vi "generate_jv_filepath.vi"(6 "Light or dark":string, 9 "Pixel":string, 10 "Cell Label":string, 11 "Data Output Folder":path) -> (2 "Scan number":string, 3 "File path":path)   [LabVIEW 2016]
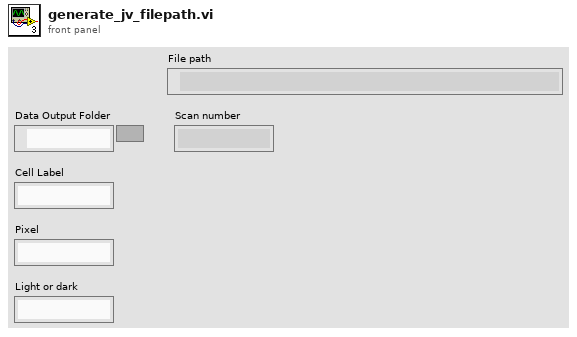
[diagram p1: front panel]
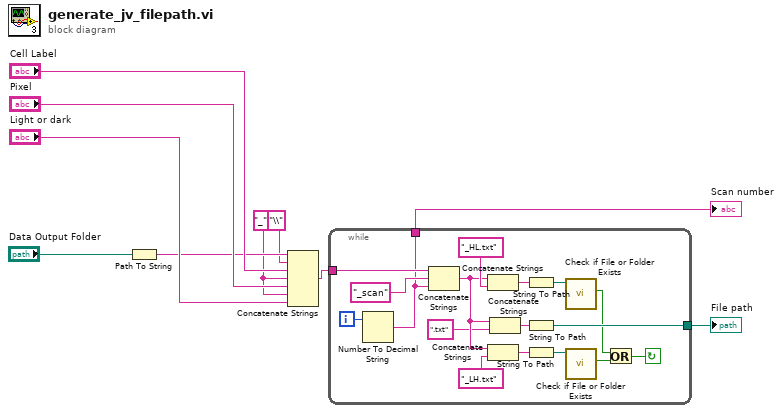
[diagram p0: block diagram]
diagram:
  w2 = "_"
  n1 = Path To String(path="Data Output Folder") -> (string=w4:string)
  n2 = Concatenate Strings(w4, "\\", "Cell Label", w2, "Pixel", w2, "Light or dark") -> (w5:string)
  n3 = while {
    tunnel: w5 -> [w27]
    tunnel: [w24] -> w9
    tunnel: [w18] -> w1
    i -> [w23]
    stop <- w14 continue-if-true
    n4 = Number To Decimal String(number=w23) -> (decimal integer string=w24:string)  [unwired: 1 in]
    n5 = Concatenate Strings(w27, "_scan", w24) -> (w13:string)
    n6 = Concatenate Strings(w13, "_HL.txt") -> (w22:string)
    n7 = Concatenate Strings(w13, "_LH.txt") -> (w19:string)
    n8 = Concatenate Strings(w13, ".txt" ("string")) -> (w11:string)
    n9 = String To Path(string=w22) -> (path=w25:path)
    n10 = String To Path(string=w11) -> (path=w18:path)
    n11 = String To Path(string=w19) -> (path=w17:path)
    n12 = call <vilib>:"Check if File or Folder Exists.vi"("path"=w25) -> ("file or folder exists?"=w15:bool)  [unwired: 8 in, 2 out]
    n13 = call <vilib>:"Check if File or Folder Exists.vi"("path"=w17) -> ("file or folder exists?"=w16:bool)  [unwired: 8 in, 2 out]
    n14 = Or(x=w15, y=w16) -> (x .or. y?=w14:bool)
  }
  "Scan number" <- w9
  "File path" <- w1
